vi "pl1000UnitInfo.vi"(8 "error in (no error)":errorcluster, 11 "pl1000 handle":i16) -> (0 "error out":errorcluster, 2 "UnitInfo":T1, 3 "pl1000 handle out":i16)   [LabVIEW 2010]
uses:
  pl1000.dll
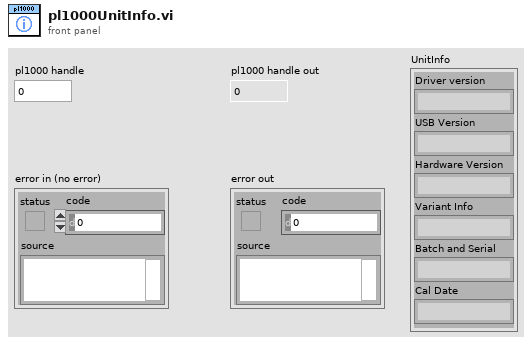
[diagram p1: front panel]
types:
  T1 = cluster{"Driver version":string, "USB Version":string, "Hardware Version":string, "Variant Info":string, "Batch and Serial":string, "Cal Date":string, "[6]":string, "[7]":string, "[8]":string}
  T2 = cluster{"status":bool, "code":u32, "source":string}
  T3 = cluster{"[0]":string, "[1]":string, "[2]":string, "[3]":string, "[4]":string, "[5]":string, "[6]":string, "[7]":string, "[8]":string}
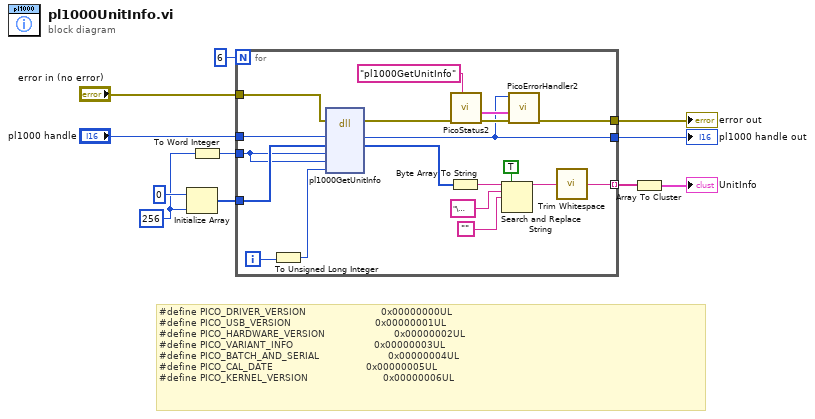
[diagram p0: block diagram]
diagram:
  w9 = 256 ("dimension size")
  # "#define\tPICO_DRIVER_VERSION                         0x00000000UL\n#define\tPICO_USB_VERSION                            0x00000001UL\n#define\tPICO_HARDWARE_VERSION                       0x00000002UL\n#define\tPICO_VARIANT_INFO                           0x00000003UL\n#define\tPICO_BATCH_AND_SERIAL                       0x00000004UL\n#define\tPICO_CAL_DATE                               0x00000005UL\n#define\tPICO_KERNEL_VERSION                         0x00000006UL"
  n1 = Initialize Array(u8 0 ("U8"), w9) -> (w11:u8[])
  n2 = To Word Integer(number=w9) -> (16bit integer=w1:i16)
  n3 = for {
    N: 6 -> [_]
    tunnel: w11 -> [w24]
    tunnel: [w23] -> w7 mode=indexing
    tunnel: "error in (no error)" -> [w20]
    tunnel: [w14] -> w3
    tunnel: "pl1000 handle" -> [w19]
    tunnel: [w12] -> w4
    tunnel: w1 -> [w18]
    i -> [w22]
    n4 = To Unsigned Long Integer(number=w22) -> (unsigned 32bit integer=w21:u32)
    n5 = dll-call lib="pl1000.dll" fn="pl1000GetUnitInfo"(error in=w20, "Handle"=w19, "String"=w24, "StringLength"=w18, "RequiredSize"=w18, "PICO_INFO"=w21) -> (error out=w15:errorcluster, "Handle"=w12:i16, "String"=w25:u8[])  [unwired: 6 in, 1 out]
    n6 = Byte Array To String(unsigned byte array=w25) -> (string=w29:string)
    n7 = call "PicoStatus2.vi"("PICO source"="pl1000GetUnitInfo", "Error in"=w15) -> ("error out"=w13:errorcluster, "PICO_STATUS out"=w17:T2)  [unwired: 6 in]
    n8 = Search and Replace String(replace all?=TRUE ("replace all? (F)"), input string=w29, search string="\u0000", replace string="") -> (result string=w28:string)  [unwired: 4 in, 3 out]
    n9 = call "PicoErrorHandler2.vi"("error in (no error)"=w13, "PICO_STATUS in"=w17, "handle In"=w12) -> ("error out"=w14:errorcluster)  [unwired: 8 in]
    n10 = call <vilib>:"Trim Whitespace.vi"("string"=w28) -> ("trimmed string"=w23:string)  [unwired: 1 in]
  }
  "pl1000 handle out" <- w4
  "error out" <- w3
  n11 = Array To Cluster(array=w7) -> (cluster=→"UnitInfo":T3)
